vi "TIFF_PreHeaderInfo.vi"(8 "error in (no error)":errorcluster) -> (0 "error out":errorcluster)   [LabVIEW 2016]
uses:
  GV/SC5_Variables.vi
  lib/Halloween/SaveTIFF/Class/Tag/IFD_Tag.lvclass
  1)Acquisition/GV/ACQ_GV.vi
  Ctl/Device Type.ctl
  2)Ref ROI/GV/ROI_GV.vi
  Scanner(x64)_LLB/Scanner/Ctl/INI_Cmd.ctl
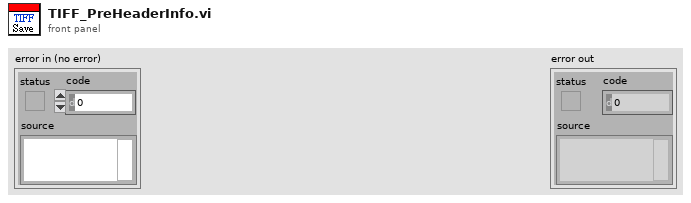
[diagram p1: front panel]
types:
  T1 = typedef "INI_Cmd.ctl" = enum16{"Flush", "Input", "Output"}
  T2 = enum16{"Undefined(DO NOT USE)", "U8", "ASCII", "U16", "U32", "RATIONAL", "I8", "Undefined 8 bit", "I16", "I32", "SRATIONAL", "SGL", "DBL"}
  T3 = enum16{"Undefined(DO NOT USE)", "pixel", "inch", "cm"}
  T4 = enum8{"FVB", "Multi Track", "Random Track", "Single Track", "2D"}
  T5 = enum8{"Not Selected", "Absorption", "Transmission", "Subtraction"}
  T6 = enum32{"Wavelength (nm)", "Pixel", "Wavenumber (cm^-1)"}
  T7 = typedef "Device Type.ctl" = enum32{"Mightex full color CCD", "PMT", "Spectrometer", "FF-Camera", "FLIM"}
  T8 = typedef "All Parameters.ctl" = cluster{"Scanner":T9, "ROI ":T12, "Spec Header":T14, "i":i32, "ref":T16, "Stage":T17}
  T9 = typedef "Scanner Param.ctl" = cluster{"Scan Area":dbl, "X Pixel":i32, "Y Pixel":i32, "Points":i32, "X Galvo Deg":dbl, "Y Galvo Deg":dbl, "X Galvo Offset":dbl, "Y Galvo Offset":dbl, "Dwell(ms)":dbl, "Frames Dwell(s)":dbl, "Extra Pixel(all)":i32, "Extra Pixel(Return)":i32, "Objective":i32, "Total Frames":i32, "Scan Direction":bool, "Transform Method":T10, "PMT Type":enum16{"Digital", "Analog"}, "AO Array":dbl[][], "Scanned Graph":dbl[][], "Size(um)_Scanned Graph":dbl, "Ref Graph":dbl[][], "Scan Mode":T11, "Spectra Scan Graphs ":sgl[][][]}
  T10 = typedef "Transform Method.ctl" = enum16{"Flip Y", "Flip X", "Rotate Left 90", "Rotate Right 90", "Rotate 180", "AntiDiagonal Mirror", "Diagonal Mirror", "None"}
  T11 = typedef "Scan Mode.ctl" = string
  T12 = typedef "ROI.ctl" = cluster{"Scan Area":dbl, "Horizonal Pixel":i32, "Vertical Pixel":i32, "Points":i32, "Y/X Pixel":dbl, "X Galvo Deg":dbl, "Y Galvo Deg":dbl, "X Galvo Offset":dbl, "Y Galvo Offset":dbl, "ROI X Size(um)":dbl, "ROI Y Size(um)":dbl, "Size(um)_ref Graph":dbl, "UI Size_Scaned Graph":i32, "UI Size_ROI Layer":i32, "Coors1":cluster{"X":dbl, "Y":dbl}, "Coors2":cluster{"X":dbl, "Y":dbl}, "Select ROI":T13, "ROI Layer Picture":picture}
  T13 = typedef "SelectROI.ctl" = enum32{"Dot", "Line", "Square", "Rectangle", "Clr"}
  T14 = typedef "Spec Header.ctl" = cluster{"SpecName ":string, "Grating":string, "CCD.ModuleNo":string, "CCD.SerialNo":string, "Exposure (ms )":dbl, "Average":i32, "Boxcar":i32, "KineticCT (ms )":dbl, "Center":dbl, "Graph":cluster{"Y":sgl[], "X":sgl[]}, "Ref":sgl[], "Reversion":bool, "Laser(nm)":dbl, "Take REF":string, "date/time":string, "X Mode":string, "Spectra No":i32, "Scan":bool, "PixelNumber":i32, "AcqMode":T15, "CCD Type":string}
  T15 = typedef "AcqMode.ctl" = enum16{"Monitor", "Acquisition"}
  T16 = typedef "Control ref.ctl" = cluster{"Scanned Graph ref":refnum<vi>, "Ref Graph ref":refnum<vi>, "R-Spec":refnum<queue>, "R-Spec Log":refnum<queue>}
  T17 = typedef "Stage.ctl" = cluster{"Position(pulse)":i32[], "UnitSize(pulse/um)":dbl[], "Upper Limit(pulse)":i32[], "Lower Limit(pulse)":i32[], "ZeroPos(pulse)":dbl[], "COM":refnum<visa-resource-name>, "Frame#":i32, "Z-Stack Position(pulse)":dbl[], "Controller mode":T18, "Z-Stack":bool, "Z Param":T19, "Z-Stack Position(um)":dbl[], "System Name":string, "StepSize":dbl[], "UnitLabel":string[], "Reverse":i32[], "XyzrIndex":i32[], "Speed":i32[][][], "Current Position(um)":dbl[], "PosTo":refnum<vi>[], "axis ref":cluster{"x-axis":refnum<vi>, "y-axis":refnum<vi>, "z-axis":refnum<vi>, "r-axis":refnum<vi>}, "Supercontinuum":cluster{"Grating Type":string, "Amplitude":dbl, "Pulse to Half Turn":dbl, "Zeroth Order Position":dbl, "Zero Shift":dbl, "MaxWL":dbl, "MinWL":dbl}, "SIGMATECH":cluster{"ClosedLoop":bool[]}}
  T18 = typedef "ControllerMode.ctl" = enum16{"SHOT-304", "FINE-01 Gamma", "PAT-001", "SHOT-102", "FINE-503", "SHOT-602", "SHOT-702", "FC-401"}
  T19 = typedef "Z Param.ctl" = cluster{"Total Frames":i32, "Step":dbl, "Start":dbl, "End":dbl, "axis":i32}
  T20 = enum16{"big-endian, network order", "native, host order", "little-endian"}
  T21 = typedef "Cofig_SelectROI.ctl" = enum32{"Dot", "Line", "Square", "Rectangle", "Clr"}
  T22 = cluster{"Data BG":enum8{"No BG", "Not Subtracted", "Subtracted"}, "Ref BG":enum8{"No BG", "Not Subtracted", "Subtracted"}, "Data Processed":enum8{"No Ref", "Not Processed", "Processed"}, "Process Method":enum8{"Not Selected", "Absorption", "Transmission", "Subtraction"}}
  T23 = cluster{"Readout Mode":enum8{"FVB", "Multi Track", "Random Track", "Single Track", "2D"}, u8, u8, "X-Axis Unit":enum32{"Wavelength (nm)", "Pixel", "Wavenumber (cm^-1)"}}
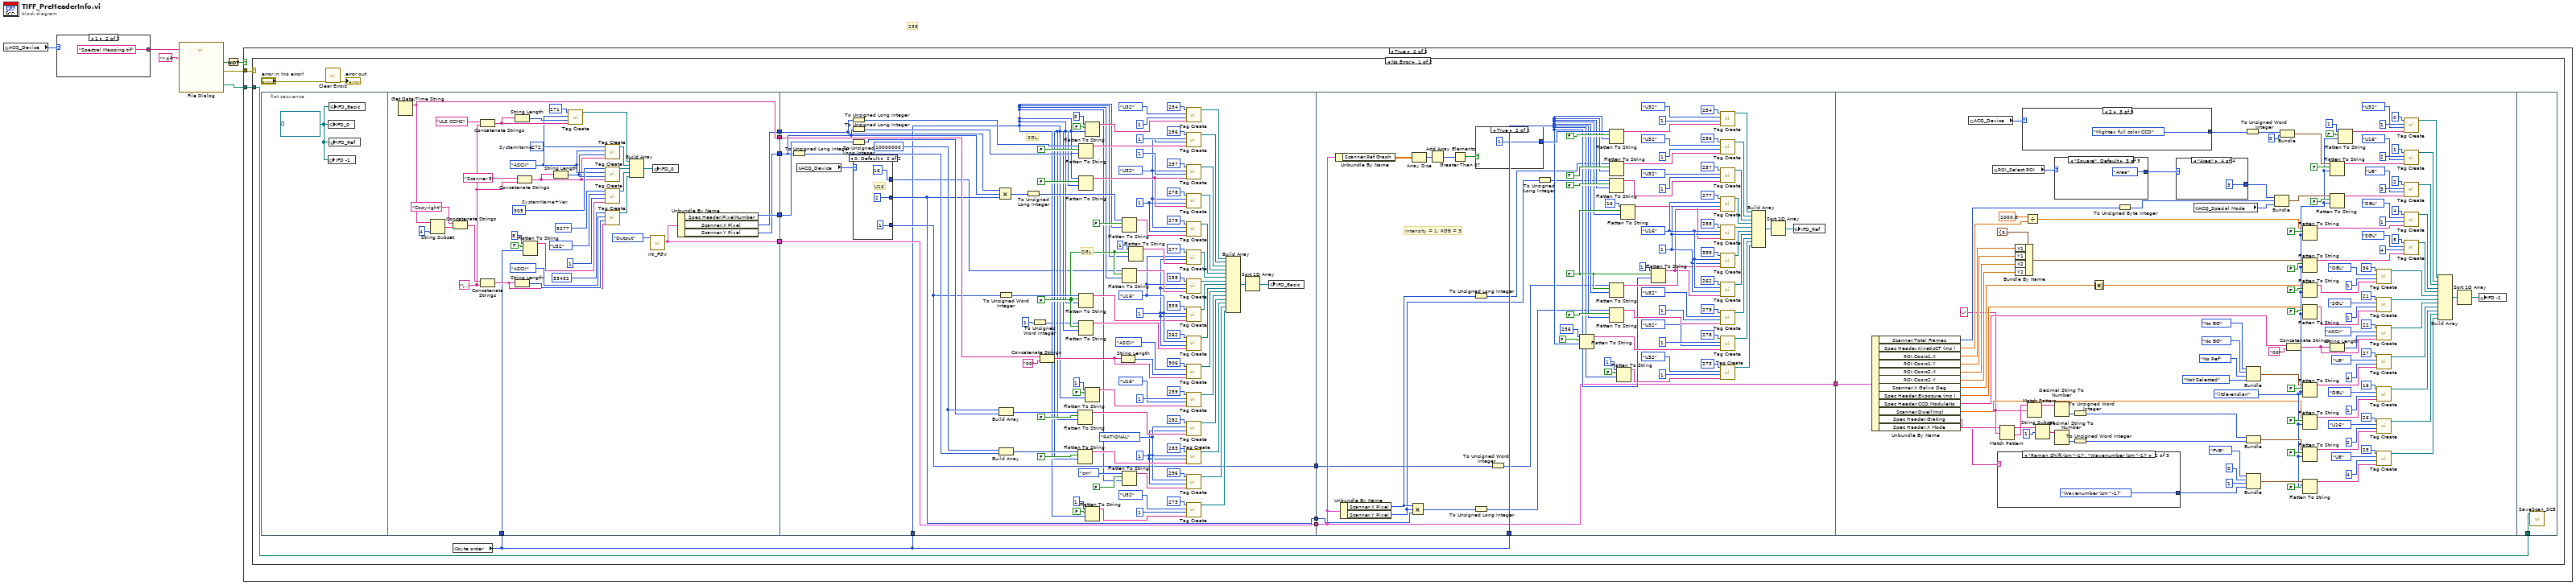
[diagram p0: block diagram]
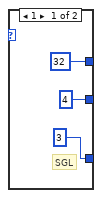
[diagram p3: hidden frame]
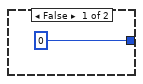
[diagram p4: hidden frame]
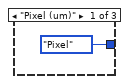
[diagram p5: hidden frame]
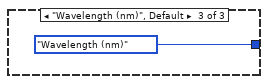
[diagram p6: hidden frame]
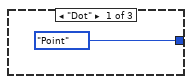
[diagram p7: hidden frame]
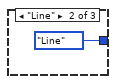
[diagram p8: hidden frame]
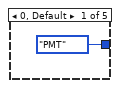
[diagram p9: hidden frame]
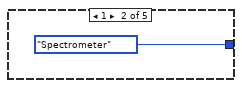
[diagram p10: hidden frame]
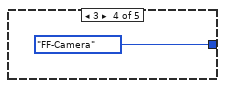
[diagram p11: hidden frame]
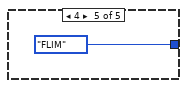
[diagram p12: hidden frame]
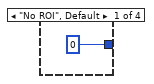
[diagram p13: hidden frame]
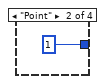
[diagram p14: hidden frame]
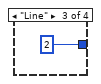
[diagram p15: hidden frame]
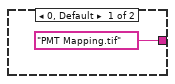
[diagram p17: hidden frame]
diagram:
  # "258"
  n1 = global read "ACQ_GV.vi" "ACQ_Device"() -> (w7:u16)
  n2 = case shown="1" w7 {
    tunnel: ["PMT Mapping.tif" ("default name") "Spectral Mapping.tif" ("default name")] -> w6
    frame 0, Default {
    }
    frame 1 {
    }
  }
  n3 = call "File Dialog"("default name"=w6, "pattern (all files)"="*.tif") -> ("selected path"=w4:path, "cancelled"=w2:bool, "error out"=w3:errorcluster)  [unwired: 10 in, 1 out]
  n4 = Not(x=w2) -> (.not. x?=w1:bool)
  n5 = case shown="True" w1 {
    tunnel: w4 -> [_ w11]
    tunnel: w3 -> [_ w10]
    frame False {
    }
    frame True {
      n6 = case shown="No Error" w10 {
        tunnel: w11 -> [w12 _]
        frame No Error {
          n7 = flat-sequence {
            tunnel: [w32] -> w24
            tunnel: [w27] -> w23
            tunnel: [w30] -> w22
            tunnel: w15 -> [w29]
            tunnel: [w28] -> w21
            tunnel: [w26] -> w20
            tunnel: w24 -> [w137]
            tunnel: w23 -> [w136]
            tunnel: w22 -> [w76]
            tunnel: [w76] -> w19
            tunnel: w15 -> [w68]
            tunnel: w21 -> [w75]
            tunnel: w20 -> [w65]
            tunnel: [w73] -> w18
            tunnel: [w72] -> w17
            tunnel: w19 -> [w171]
            tunnel: w15 -> [w179]
            tunnel: [w171] -> w16
            tunnel: w18 -> [w172]
            tunnel: w17 -> [w170]
            tunnel: w16 -> [w275]
            tunnel: w12 -> [w385]
            frame #0 {
              w25 = refnum<class "IFD_Tag.lvclass">[] [] ("IFD_0")
              n8 = global write "SC5_Variables.vi" "IFD -1"(w25) -> ()
              n9 = global write "SC5_Variables.vi" "IFD_0"(w25) -> ()
              n10 = global write "SC5_Variables.vi" "IFD_Ref"(w25) -> ()
              n11 = global write "SC5_Variables.vi" "IFD_Basic"(w25) -> ()
            }
            frame #1 {
              w43 = T2."ASCII" ("Data Type")
              w48 = u16 305  # SystemName+Ver.
              w44 = u16 272  # SystemName
              w63 = "\u0000"
              n12 = Get Date/Time String() -> (date string=w28:string)  [unwired: 3 in, 1 out]
              n13 = String Subset(string=w28, length (rest)=4 ("length (rest)")) -> (substring=w31:string)  [unwired: 1 in]
              n14 = Concatenate Strings("Copyright", w31) -> (w57:string)
              n15 = Concatenate Strings("ULS CCMS", w63) -> (w45:string)
              n16 = Concatenate Strings(w57, w63) -> (w53:string)
              n17 = String Length(string=w45) -> (length=w46:i32)
              n18 = String Length(string=w53) -> (length=w54:i32)
              n19 = Concatenate Strings("Scanner 5" ("string"), w63) -> (w41:string)
              n20 = Flatten To String(anything=u32 8, prepend array or string size? (T)=FALSE, byte order (0:big-endian, network order)=w29) -> (data string=w52:string)  [unwired: 1 in, 2 out]
              n21 = String Length(string=w41) -> (length=w42:i32)
              n22 = call "Tag Create.vi"("Data"=w45, "Data Count"=w46, "Data Type"=w43, "Tag ID"=u16 271) -> ("IFD_Tag out"=w39:refnum<class "IFD_Tag.lvclass">)  [unwired: 7 in]
              n23 = call "Tag Create.vi"("Data"=w41, "Data Count"=w42, "Data Type"=w43, "Tag ID"=w44) -> ("IFD_Tag out"=w38:refnum<class "IFD_Tag.lvclass">)  [unwired: 7 in]
              n24 = call "Tag Create.vi"("Data"=w41, "Data Count"=w42, "Data Type"=w43, "Tag ID"=w48) -> ("IFD_Tag out"=w37:refnum<class "IFD_Tag.lvclass">)  [unwired: 7 in]
              n25 = call "Tag Create.vi"("Data"=w52, "Data Count"=u32 1, "Data Type"=T2."U32", "Tag ID"=u16 5277) -> ("IFD_Tag out"=w36:refnum<class "IFD_Tag.lvclass">)  [unwired: 7 in]
              n26 = call "Tag Create.vi"("Data"=w53, "Data Count"=w54, "Data Type"=T2."ASCII", "Tag ID"=u16 33432) -> ("IFD_Tag out"=w35:refnum<class "IFD_Tag.lvclass">)  [unwired: 7 in]
              n27 = Build Array(w39, w38, w37, w36, w35) -> (w34:refnum<class "IFD_Tag.lvclass">[])
              n28 = call "INI_FGV.vi"("Cmd"=INI_Cmd."Output") -> ("Output"=w30:T8)  [unwired: 9 in, 1 out]
              n29 = global write "SC5_Variables.vi" "IFD_0"(w34) -> ()
              n30 = Unbundle By Name(w30) -> ("Spec Header.PixelNumber"=w32:i32, "Scanner.X Pixel"=w26:i32, "Scanner.Y Pixel"=w27:i32)
            }
            frame #2 {
              w145 = u32 10000000 ("Public Denominator")
              w86 = T2."RATIONAL" ("Data Type")
              w85 = u32 1 ("Data Count")
              w69 = FALSE ("prepend array or string size? (T)")
              w110 = u32 1 ("Data Count")
              w111 = T2."U16" ("Data Type")
              w123 = u32 1 ("Data Count")
              w124 = T2."U32" ("Data Type")
              # "SGL"
              # "SGL"
              n31 = To Unsigned Long Integer(number=w136) -> (unsigned 32bit integer=w139:u32)
              n32 = global read "ACQ_GV.vi" "ACQ_Device"() -> (w74:u16)
              n33 = To Unsigned Long Integer(number=w65) -> (unsigned 32bit integer=w154:u32)
              n34 = To Unsigned Long Integer(number=w136) -> (unsigned 32bit integer=w153:u32)
              n35 = To Unsigned Long Integer(number=w137) -> (unsigned 32bit integer=w140:u32)
              n36 = case shown="0, Default" w74 {
                tunnel: [4 ("x") 2 ("x")] -> w73
                tunnel: [u16 3 ("number") u16 1 ("number")] -> w72
                tunnel: [u16 32 u16 16] -> w64
                frame 1 {
                  # "SGL"
                }
                frame 0, Default {
                  # "U16"
                }
              }
              n37 = To Unsigned Word Integer(number=w72) -> (unsigned 16bit integer=w138:u16)
              n38 = Build Array(w145, w140) -> (w148:u32[])
              n39 = Build Array(w145, w139) -> (w147:u32[])
              n40 = Compound Arithmetic op=MULTIPLY(w65, w136, w73) -> (w160:i32)
              n41 = To Unsigned Long Integer(number=w160) -> (unsigned 32bit integer=w152:u32)
              n42 = To Unsigned Word Integer(number=u16 1) -> (unsigned 16bit integer=w67:u16)
              n43 = Concatenate Strings(w75, "00" ("string")) -> (w105:string)
              n44 = Flatten To String(anything=w148, prepend array or string size? (T)=FALSE, byte order (0:big-endian, network order)=w68) -> (data string=w92:string)  [unwired: 1 in, 2 out]
              n45 = Flatten To String(anything=w147, prepend array or string size? (T)=FALSE, byte order (0:big-endian, network order)=w68) -> (data string=w89:string)  [unwired: 1 in, 2 out]
              n46 = Flatten To String(anything=w154, prepend array or string size? (T)=FALSE, byte order (0:big-endian, network order)=w68) -> (data string=w133:string)  [unwired: 1 in, 2 out]
              n47 = Flatten To String(anything=w153, prepend array or string size? (T)=FALSE, byte order (0:big-endian, network order)=w68) -> (data string=w127:string)  [unwired: 1 in, 2 out]
              n48 = Flatten To String(anything=w138, prepend array or string size? (T)=w69, byte order (0:big-endian, network order)=w68) -> (data string=w71:string)  [unwired: 1 in, 2 out]
              n49 = Flatten To String(anything=w67, prepend array or string size? (T)=w69, byte order (0:big-endian, network order)=w68) -> (data string=w70:string)  [unwired: 1 in, 2 out]
              n50 = Flatten To String(anything=u32 0, prepend array or string size? (T)=FALSE, byte order (0:big-endian, network order)=w68) -> (data string=w100:string)  [unwired: 1 in, 2 out]
              n51 = Flatten To String(anything=u16 1, prepend array or string size? (T)=FALSE, byte order (0:big-endian, network order)=w68) -> (data string=w95:string)  [unwired: 1 in, 2 out]
              n52 = Flatten To String(anything=u32 1, prepend array or string size? (T)=FALSE, byte order (0:big-endian, network order)=w68) -> (data string=w79:string)  [unwired: 1 in, 2 out]
              n53 = String Length(string=w105) -> (length=w106:i32)
              n54 = Flatten To String(anything=w152, prepend array or string size? (T)=FALSE, byte order (0:big-endian, network order)=w68) -> (data string=w122:string)  [unwired: 1 in, 2 out]
              n55 = Flatten To String(anything=w64, prepend array or string size? (T)=w69, byte order (0:big-endian, network order)=w68) -> (data string=w116:string)  [unwired: 1 in, 2 out]
              n56 = Flatten To String(anything=T3."cm" ("Basic Unit"), prepend array or string size? (T)=FALSE, byte order (0:big-endian, network order)=w68) -> (data string=w84:string)  [unwired: 1 in, 2 out]
              n57 = Flatten To String(anything=u16 1, prepend array or string size? (T)=w69, byte order (0:big-endian, network order)=w68) -> (data string=w119:string)  [unwired: 1 in, 2 out]
              n58 = call "Tag Create.vi"("Data"=w100, "Data Count"=u32 1, "Data Type"=T2."U32", "Tag ID"=u16 254) -> ("IFD_Tag out"=w99:refnum<class "IFD_Tag.lvclass">)  [unwired: 7 in]
              n59 = call "Tag Create.vi"("Data"=w133, "Data Count"=u32 1, "Data Type"=w124, "Tag ID"=u16 256) -> ("IFD_Tag out"=w132:refnum<class "IFD_Tag.lvclass">)  [unwired: 7 in]
              n60 = call "Tag Create.vi"("Data"=w127, "Data Count"=u32 1, "Data Type"=w124, "Tag ID"=u16 257) -> ("IFD_Tag out"=w129:refnum<class "IFD_Tag.lvclass">)  [unwired: 7 in]
              n61 = call "Tag Create.vi"("Data"=w127, "Data Count"=w123, "Data Type"=w124, "Tag ID"=u16 278) -> ("IFD_Tag out"=w126:refnum<class "IFD_Tag.lvclass">)  [unwired: 7 in]
              n62 = call "Tag Create.vi"("Data"=w122, "Data Count"=w123, "Data Type"=w124, "Tag ID"=u16 279) -> ("IFD_Tag out"=w121:refnum<class "IFD_Tag.lvclass">)  [unwired: 7 in]
              n63 = call "Tag Create.vi"("Data"=w119, "Data Count"=w110, "Data Type"=w111, "Tag ID"=u16 277) -> ("IFD_Tag out"=w118:refnum<class "IFD_Tag.lvclass">)  [unwired: 7 in]
              n64 = call "Tag Create.vi"("Data"=w116, "Data Count"=w110, "Data Type"=w111, "Tag ID"=u16 258) -> ("IFD_Tag out"=w115:refnum<class "IFD_Tag.lvclass">)  [unwired: 7 in]
              n65 = call "Tag Create.vi"("Data"=w71, "Data Count"=w110, "Data Type"=w111, "Tag ID"=u16 339) -> ("IFD_Tag out"=w113:refnum<class "IFD_Tag.lvclass">)  [unwired: 7 in]
              n66 = call "Tag Create.vi"("Data"=w70, "Data Count"=w110, "Data Type"=w111, "Tag ID"=u16 262) -> ("IFD_Tag out"=w109:refnum<class "IFD_Tag.lvclass">)  [unwired: 7 in]
              n67 = call "Tag Create.vi"("Data"=w105, "Data Count"=w106, "Data Type"=T2."ASCII", "Tag ID"=u16 306) -> ("IFD_Tag out"=w104:refnum<class "IFD_Tag.lvclass">)  [unwired: 7 in]
              n68 = call "Tag Create.vi"("Data"=w95, "Data Count"=u32 1, "Data Type"=T2."U16", "Tag ID"=u16 259) -> ("IFD_Tag out"=w94:refnum<class "IFD_Tag.lvclass">)  [unwired: 7 in]
              n69 = call "Tag Create.vi"("Data"=w92, "Data Count"=w85, "Data Type"=w86, "Tag ID"=u16 282) -> ("IFD_Tag out"=w91:refnum<class "IFD_Tag.lvclass">)  [unwired: 7 in]
              n70 = call "Tag Create.vi"("Data"=w89, "Data Count"=w85, "Data Type"=w86, "Tag ID"=u16 283) -> ("IFD_Tag out"=w88:refnum<class "IFD_Tag.lvclass">)  [unwired: 7 in]
              n71 = call "Tag Create.vi"("Data"=w84, "Data Count"=w85, "Data Type"=w86, "Tag ID"=u16 296) -> ("IFD_Tag out"=w83:refnum<class "IFD_Tag.lvclass">)  [unwired: 7 in]
              n72 = call "Tag Create.vi"("Data"=w79, "Data Count"=u32 1, "Data Type"=T2."U32", "Tag ID"=u16 273) -> ("IFD_Tag out"=w78:refnum<class "IFD_Tag.lvclass">)  [unwired: 7 in]
              n73 = Build Array(w99, w132, w129, w126, w121, w118, w115, w113, w109, w104, w94, w91, w88, w83, w78) -> (w155:refnum<class "IFD_Tag.lvclass">[])
              n74 = Sort 1D Array(array=w155) -> (sorted array=w77:refnum<class "IFD_Tag.lvclass">[])
              n75 = global write "SC5_Variables.vi" "IFD_Basic"(w77) -> ()
            }
            frame #3 {
              w219 = FALSE ("prepend array or string size? (T)")
              w222 = u32 1 ("Data Count")
              w223 = T2."U16" ("Data Type")
              # "Intensity = 1, RGB = 3"
              n76 = Unbundle By Name(w171) -> ("Scanner.Ref Graph"=w184:dbl[][])
              n77 = Unbundle By Name(w171) -> ("Scanner.X Pixel"=w176:i32, "Scanner.Y Pixel"=w174:i32)
              n78 = Array Size(array=w184) -> (size(s)=w183:i32[])
              n79 = Compound Arithmetic op=MULTIPLY(w176, w174, w172) -> (w205:i32)
              n80 = Add Array Elements(numeric array=w183) -> (sum=w182:i32)
              n81 = Greater Than 0?(x=w182) -> (x > 0?=w181:bool)
              n82 = To Unsigned Long Integer(number=w176) -> (unsigned 32bit integer=w175:u32)
              n83 = To Unsigned Long Integer(number=w205) -> (unsigned 32bit integer=w177:u32)
              n84 = case shown="True" w181 {
                tunnel: [u32 0 u32 1] -> w240
                frame False {
                }
                frame True {
                }
              }
              n85 = To Unsigned Word Integer(number=w170) -> (unsigned 16bit integer=w178:u16)
              n86 = To Unsigned Long Integer(number=w174) -> (unsigned 32bit integer=w173:u32)
              n87 = Flatten To String(anything=u32 256, prepend array or string size? (T)=FALSE, byte order (0:big-endian, network order)=w179) -> (data string=w200:string)  [unwired: 1 in, 2 out]
              n88 = Flatten To String(anything=w240, prepend array or string size? (T)=FALSE, byte order (0:big-endian, network order)=w179) -> (data string=w185:string)  [unwired: 1 in, 2 out]
              n89 = Flatten To String(anything=w175, prepend array or string size? (T)=FALSE, byte order (0:big-endian, network order)=w179) -> (data string=w234:string)  [unwired: 1 in, 2 out]
              n90 = Flatten To String(anything=w173, prepend array or string size? (T)=FALSE, byte order (0:big-endian, network order)=w179) -> (data string=w229:string)  [unwired: 1 in, 2 out]
              n91 = Flatten To String(anything=w178, prepend array or string size? (T)=w219, byte order (0:big-endian, network order)=w179) -> (data string=w217:string)  [unwired: 1 in, 2 out]
              n92 = Flatten To String(anything=w177, prepend array or string size? (T)=FALSE, byte order (0:big-endian, network order)=w179) -> (data string=w208:string)  [unwired: 1 in, 2 out]
              n93 = Flatten To String(anything=u32 1, prepend array or string size? (T)=FALSE, byte order (0:big-endian, network order)=w179) -> (data string=w192:string)  [unwired: 1 in, 2 out]
              n94 = Flatten To String(anything=u16 16, prepend array or string size? (T)=w219, byte order (0:big-endian, network order)=w179) -> (data string=w218:string)  [unwired: 1 in, 2 out]
              n95 = Flatten To String(anything=u16 1, prepend array or string size? (T)=w219, byte order (0:big-endian, network order)=w179) -> (data string=w216:string)  [unwired: 1 in, 2 out]
              n96 = call "Tag Create.vi"("Data"=w185, "Data Count"=u32 1, "Data Type"=T2."U32", "Tag ID"=u16 254) -> ("IFD_Tag out"=w189:refnum<class "IFD_Tag.lvclass">)  [unwired: 7 in]
              n97 = call "Tag Create.vi"("Data"=w234, "Data Count"=u32 1, "Data Type"=T2."U32", "Tag ID"=u16 256) -> ("IFD_Tag out"=w236:refnum<class "IFD_Tag.lvclass">)  [unwired: 7 in]
              n98 = call "Tag Create.vi"("Data"=w229, "Data Count"=u32 1, "Data Type"=T2."U32", "Tag ID"=u16 257) -> ("IFD_Tag out"=w228:refnum<class "IFD_Tag.lvclass">)  [unwired: 7 in]
              n99 = call "Tag Create.vi"("Data"=w216, "Data Count"=w222, "Data Type"=w223, "Tag ID"=u16 277) -> ("IFD_Tag out"=w215:refnum<class "IFD_Tag.lvclass">)  [unwired: 7 in]
              n100 = call "Tag Create.vi"("Data"=w218, "Data Count"=w222, "Data Type"=w223, "Tag ID"=u16 258) -> ("IFD_Tag out"=w214:refnum<class "IFD_Tag.lvclass">)  [unwired: 7 in]
              n101 = call "Tag Create.vi"("Data"=w217, "Data Count"=w222, "Data Type"=w223, "Tag ID"=u16 339) -> ("IFD_Tag out"=w213:refnum<class "IFD_Tag.lvclass">)  [unwired: 7 in]
              n102 = call "Tag Create.vi"("Data"=w216, "Data Count"=w222, "Data Type"=w223, "Tag ID"=u16 262) -> ("IFD_Tag out"=w212:refnum<class "IFD_Tag.lvclass">)  [unwired: 7 in]
              n103 = call "Tag Create.vi"("Data"=w208, "Data Count"=u32 1, "Data Type"=T2."U32", "Tag ID"=u16 279) -> ("IFD_Tag out"=w207:refnum<class "IFD_Tag.lvclass">)  [unwired: 7 in]
              n104 = call "Tag Create.vi"("Data"=w200, "Data Count"=u32 1, "Data Type"=T2."U32", "Tag ID"=u16 278) -> ("IFD_Tag out"=w198:refnum<class "IFD_Tag.lvclass">)  [unwired: 7 in]
              n105 = call "Tag Create.vi"("Data"=w192, "Data Count"=u32 1, "Data Type"=T2."U32", "Tag ID"=u16 273) -> ("IFD_Tag out"=w194:refnum<class "IFD_Tag.lvclass">)  [unwired: 7 in]
              n106 = Build Array(w189, w236, w228, w215, w214, w213, w212, w207, w198, w194) -> (w197:refnum<class "IFD_Tag.lvclass">[])
              n107 = Sort 1D Array(array=w197) -> (sorted array=w180:refnum<class "IFD_Tag.lvclass">[])
              n108 = global write "SC5_Variables.vi" "IFD_Ref"(w180) -> ()
            }
            frame #4 {
              w254 = "-" ("regular expression")
              w277 = T20."little-endian" ("byte order")
              n109 = Unbundle By Name(w275) -> ("Scanner.Total Frames"=w269:i32, "Spec Header.KineticCT (ms )"=w268:dbl, "ROI.Coors1.X"=w265:dbl, "ROI.Coors1.Y"=w264:dbl, "ROI.Coors2.X"=w263:dbl, "ROI.Coors2.Y"=w262:dbl, "Scanner.X Galvo Deg"=w261:dbl, "Spec Header.Exposure (ms )"=w259:dbl, "Spec Header.CCD.ModuleNo"=w258:string, "Scanner.Dwell(ms)"=w257:dbl, "Spec Header.Grating"=w253:string, "Spec Header.X Mode"=w245:string)
              n110 = global read "ACQ_GV.vi" "ACQ_Device"() -> (w274:u16)
              n111 = global read "ROI_GV.vi" "ROI_Select ROI"() -> (w272:T21)
              n112 = case shown="\"Raman Shift (cm^-1)\", \"Wavenumber (cm^-1)\"" w245 {
                tunnel: [T6."Pixel" ("X-Axis Unit") T6."Wavenumber (cm^-1)" ("X-Axis Unit") T6."Wavelength (nm)" ("X-Axis Unit")] -> w244
                frame "Pixel (um)" {
                }
                frame "Raman Shift (cm^-1)", "Wavenumber (cm^-1)" {
                }
                frame "Wavelength (nm)", Default {
                }
              }
              n113 = Match Pattern(string=w253, regular expression=w254) -> (before substring=w249:string, after substring=w255:string)  [unwired: 1 in, 2 out]
              n114 = Bundle By Name(cluster=cluster{"X1":sgl, "X2":sgl, "Y1":sgl, "Y2":sgl} {"X1"=0.0, "X2"=0.0, "Y1"=0.0, "Y2"=0.0} ("ROI"), "X1"=w265, "Y1"=w264, "X2"=w263, "Y2"=w262) -> (w335:cluster{"X1":sgl, "X2":sgl, "Y1":sgl, "Y2":sgl})
              n115 = case shown="2" w274 {
                tunnel: [Device_Type."PMT" ("Scanning Instrument") Device_Type."Spectrometer" ("Scanning Instrument") Device_Type."Mightex full color CCD" ("Scanning Instrument") Device_Type."FF-Camera" ("Scanning Instrument") Device_Type."FLIM" ("Scanning Instrument")] -> w273
                frame 0, Default {
                }
                frame 1 {
                }
                frame 2 {
                }
                frame 3 {
                }
                frame 4 {
                }
              }
              n116 = Divide(x=1000.0, y=w268) -> (x/y=w266:dbl)
              n117 = Match Pattern(string=w255, regular expression=w254) -> (before substring=w252:string)  [unwired: 1 in, 3 out]
              n118 = String Subset(string=w249, offset (0)=1) -> (substring=w247:string)  [unwired: 1 in]
              n119 = case shown="\"Square\", Default" w272 {
                tunnel: [enum32{"No ROI", "Point", "Line", "Area"}."Point" ("ROI Type") enum32{"No ROI", "Point", "Line", "Area"}."Line" ("ROI Type") enum32{"No ROI", "Point", "Line", "Area"}."Area" ("ROI Type")] -> w271
                frame "Dot" {
                }
                frame "Line" {
                }
                frame "Square", Default {
                }
              }
              n120 = Decimal String To Number(string=w252) -> (number=w251:i32)  [unwired: 2 in, 1 out]
              n121 = Decimal String To Number(string=w247) -> (number=w248:i32)  [unwired: 2 in, 1 out]
              n122 = To Unsigned Word Integer(number=w251) -> (unsigned 16bit integer=w256:u16)
              n123 = To Unsigned Word Integer(number=w248) -> (unsigned 16bit integer=w246:u16)
              n124 = Absolute Value(x=w261) -> (abs(x)=w260:dbl)
              n125 = To Unsigned Byte Integer(number=w269) -> (unsigned 8bit integer=w348:u8)
              n126 = case shown="\"Area\"" w271 {
                tunnel: [u8 0 u8 1 u8 2 u8 3] -> w349
                frame "No ROI", Default {
                }
                frame "Point" {
                }
                frame "Line" {
                }
                frame "Area" {
                }
              }
              n127 = global read "ACQ_GV.vi" "ACQ_Special Mode"() -> (w270:u16)
              n128 = To Unsigned Word Integer(number=w273) -> (unsigned 16bit integer=w288:u16)
              n129 = Bundle("Data BG"=enum8{"No BG", "Not Subtracted", "Subtracted"}."No BG", "Ref BG"=enum8{"No BG", "Not Subtracted", "Subtracted"}."No BG", "Data Processed"=enum8{"No Ref", "Not Processed", "Processed"}."No Ref", "Process Method"=T5."Not Selected") -> (w308:T22)  [unwired: 1 in]
              n130 = Bundle(w256, w246) -> (w294:cluster{u16, u16})  [unwired: 1 in]
              n131 = Bundle("Readout Mode"=T4."FVB", u8 0, u8 1, "X-Axis Unit"=w244) -> (w278:T23)  [unwired: 1 in]
              n132 = Bundle(w349, w348, "ACQ_Special Mode"=w270) -> (w347:cluster{u8, u8, "ACQ_Special Mode":u16})  [unwired: 1 in]
              n133 = Bundle(w288, u16 0) -> (w357:cluster{u16, u16})  [unwired: 1 in]
              n134 = Concatenate Strings(w258, "00" ("string")) -> (w319:string)
              n135 = Flatten To String(anything=w266, prepend array or string size? (T)=FALSE, byte order (0:big-endian, network order)=w277) -> (data string=w342:string)  [unwired: 1 in, 2 out]
              n136 = Flatten To String(anything=w335, prepend array or string size? (T)=FALSE, byte order (0:big-endian, network order)=w277) -> (data string=w337:string)  [unwired: 1 in, 2 out]
              n137 = Flatten To String(anything=w260, prepend array or string size? (T)=FALSE, byte order (0:big-endian, network order)=w277) -> (data string=w329:string)  [unwired: 1 in, 2 out]
              n138 = Flatten To String(anything=w259, prepend array or string size? (T)=FALSE, byte order (0:big-endian, network order)=w277) -> (data string=w324:string)  [unwired: 1 in, 2 out]
              n139 = Flatten To String(anything=w308, prepend array or string size? (T)=FALSE, byte order (0:big-endian, network order)=w277) -> (data string=w307:string)  [unwired: 1 in, 2 out]
              n140 = Flatten To String(anything=w257, prepend array or string size? (T)=FALSE, byte order (0:big-endian, network order)=w277) -> (data string=w301:string)  [unwired: 1 in, 2 out]
              n141 = Flatten To String(anything=w294, prepend array or string size? (T)=FALSE, byte order (0:big-endian, network order)=w277) -> (data string=w295:string)  [unwired: 1 in, 2 out]
              n142 = Flatten To String(anything=w278, prepend array or string size? (T)=FALSE, byte order (0:big-endian, network order)=w277) -> (data string=w283:string)  [unwired: 1 in, 2 out]
              n143 = Flatten To String(anything=w357, prepend array or string size? (T)=FALSE, byte order (0:big-endian, network order)=w277) -> (data string=w356:string)  [unwired: 1 in, 2 out]
              n144 = Flatten To String(anything=w347, prepend array or string size? (T)=FALSE, byte order (0:big-endian, network order)=w277) -> (data string=w350:string)  [unwired: 1 in, 2 out]
              n145 = String Length(string=w319) -> (length=w318:i32)
              n146 = Flatten To String(anything=u32 1, prepend array or string size? (T)=FALSE, byte order (0:big-endian, network order)=w277) -> (data string=w364:string)  [unwired: 1 in, 2 out]
              n147 = call "Tag Create.vi"("Data"=w329, "Data Count"=u32 1, "Data Type"=T2."DBL", "Tag ID"=u16 36) -> ("IFD_Tag out"=w333:refnum<class "IFD_Tag.lvclass">)  [unwired: 7 in]
              n148 = call "Tag Create.vi"("Data"=w324, "Data Count"=u32 1, "Data Type"=T2."SGL", "Tag ID"=u16 21) -> ("IFD_Tag out"=w323:refnum<class "IFD_Tag.lvclass">)  [unwired: 7 in]
              n149 = call "Tag Create.vi"("Data"=w319, "Data Count"=w318, "Data Type"=T2."ASCII", "Tag ID"=u16 22) -> ("IFD_Tag out"=w317:refnum<class "IFD_Tag.lvclass">)  [unwired: 7 in]
              n150 = call "Tag Create.vi"("Data"=w307, "Data Count"=u32 4, "Data Type"=T2."U8", "Tag ID"=u16 27) -> ("IFD_Tag out"=w306:refnum<class "IFD_Tag.lvclass">)  [unwired: 7 in]
              n151 = call "Tag Create.vi"("Data"=w301, "Data Count"=u32 1, "Data Type"=T2."DBL", "Tag ID"=u16 16) -> ("IFD_Tag out"=w300:refnum<class "IFD_Tag.lvclass">)  [unwired: 7 in]
              n152 = call "Tag Create.vi"("Data"=w295, "Data Count"=u32 2, "Data Type"=T2."U16", "Tag ID"=u16 26) -> ("IFD_Tag out"=w293:refnum<class "IFD_Tag.lvclass">)  [unwired: 7 in]
              n153 = call "Tag Create.vi"("Data"=w283, "Data Count"=u32 4, "Data Type"=T2."U8", "Tag ID"=u16 23) -> ("IFD_Tag out"=w282:refnum<class "IFD_Tag.lvclass">)  [unwired: 7 in]
              n154 = call "Tag Create.vi"("Data"=w364, "Data Count"=u32 1, "Data Type"=T2."U32", "Tag ID"=u16 0) -> ("IFD_Tag out"=w363:refnum<class "IFD_Tag.lvclass">)  [unwired: 7 in]
              n155 = call "Tag Create.vi"("Data"=w356, "Data Count"=u32 2, "Data Type"=T2."U16", "Tag ID"=u16 1) -> ("IFD_Tag out"=w355:refnum<class "IFD_Tag.lvclass">)  [unwired: 7 in]
              n156 = call "Tag Create.vi"("Data"=w350, "Data Count"=u32 3, "Data Type"=T2."U8", "Tag ID"=u16 2) -> ("IFD_Tag out"=w346:refnum<class "IFD_Tag.lvclass">)  [unwired: 7 in]
              n157 = call "Tag Create.vi"("Data"=w342, "Data Count"=u32 1, "Data Type"=T2."DBL", "Tag ID"=u16 4) -> ("IFD_Tag out"=w341:refnum<class "IFD_Tag.lvclass">)  [unwired: 7 in]
              n158 = call "Tag Create.vi"("Data"=w337, "Data Count"=u32 4, "Data Type"=T2."SGL", "Tag ID"=u16 5) -> ("IFD_Tag out"=w334:refnum<class "IFD_Tag.lvclass">)  [unwired: 7 in]
              n159 = Build Array(w363, w355, w346, w341, w334, w333, w323, w317, w306, w300, w293, w282) -> (w289:refnum<class "IFD_Tag.lvclass">[])
              n160 = Sort 1D Array(array=w289) -> (sorted array=w276:refnum<class "IFD_Tag.lvclass">[])
              n161 = global write "SC5_Variables.vi" "IFD -1"(w276) -> ()
            }
            frame #5 {
              n162 = call "SaveScan_SC5.vi"("selected path"=w385) -> ()  [unwired: 11 in]
            }
          }
          n163 = call <vilib>:"Clear Errors.vi"("error in (no error)"="error in (no error)") -> ("error out"=→"error out":errorcluster)  [unwired: 5 in, 1 out]
          n164 = global read "SC5_Variables.vi" "byte order"() -> (w15:T20)
        }
        frame Error {
        }
      }
    }
  }
